vi "get_and_insert_SN.vi"(8 "error in (no error)":errorcluster, 10 "read buffer in":string, 11 "VISA Refnum in":refnum<visa-resource-name>) -> (0 "error out":errorcluster, 2 "read buffer out":string, 3 "VISA Refnum out":refnum<visa-resource-name>)   [LabVIEW 2015]
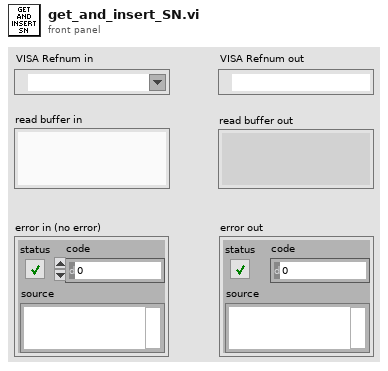
[diagram p1: front panel]
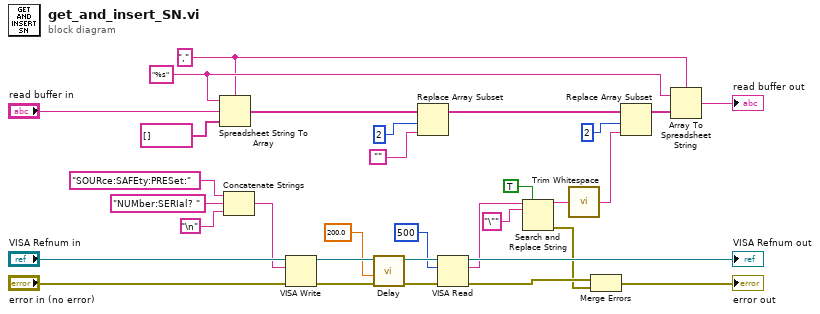
[diagram p0: block diagram]
diagram:
  w29 = "," ("delimiter (Tab)")
  w30 = "%s" ("format string")
  n1 = Spreadsheet String To Array(delimiter (Tab)=w29, format string=w30, spreadsheet string="read buffer in", array type (2D Dbl)=string[] []) -> (array=w5:string[])
  n2 = Concatenate Strings("SOURce:SAFEty:PRESet:", "NUMber:SERIal? ", "\n") -> (w12:string)
  n3 = VISA Write(VISA resource name="VISA Refnum in", write buffer=w12, error in (no error)="error in (no error)") -> (VISA resource name out=w31:refnum<visa-resource-name>, error out=w9:errorcluster)  [unwired: 1 out]
  n4 = call "Delay.vi"("error in (no error)"=w9, "milliseconds to wait"=200.0) -> ("error out"=w10:errorcluster)  [unwired: 9 in]
  n5 = Replace Array Subset(array=w5, new element="", index=2) -> (w4:string[])
  n6 = VISA Read(VISA resource name=w31, byte count=u32 500, error in (no error)=w10) -> (VISA resource name out=→"VISA Refnum out":refnum<visa-resource-name>, read buffer=w13:string, error out=w24:errorcluster)  [unwired: 1 out]
  n7 = Search and Replace String(replace all?=TRUE ("replace all? (F)"), input string=w13, search string="\"" ("substring (\"\")")) -> (result string=w22:string, error out=w6:errorcluster)  [unwired: 5 in, 2 out]
  n8 = call <vilib>:"Trim Whitespace.vi"("string"=w22) -> ("trimmed string"=w28:string)  [unwired: 1 in]
  n9 = Merge Errors(w24, w6) -> (→"error out":errorcluster)
  n10 = Replace Array Subset(array=w4, new element=w28, index=2) -> (w26:string[])
  n11 = Array To Spreadsheet String(delimiter (Tab)=w29, array=w26, 3:w30) -> (spreadsheet string=→"read buffer out":string)
